vi "Close Instrument.vi"(8 "error in (no error)":errorcluster, 11 "Example Instrument in":refnum<class "LevyLab Instrument.lvclass">) -> (0 "error out":errorcluster, 3 "Example Instrument out":refnum<class "LevyLab Instrument.lvclass">)   [LabVIEW 2016, in "LevyLab Instrument.lvclass"]
uses:
  LevyLab Instrument.lvclass
  SMOs/Instrument/Instrument.lvclass
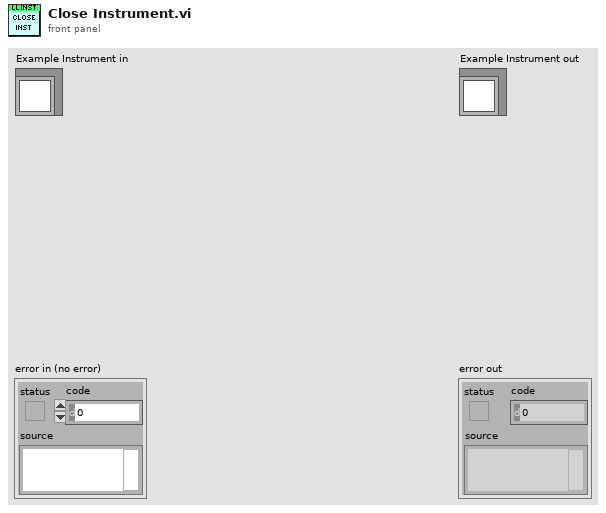
[diagram p1: front panel]
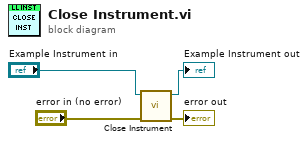
[diagram p0: block diagram]
diagram:
  n1 = call-parent "Close Instrument.vi"("error in (no error)"="error in (no error)", "Instrument in"="Example Instrument in") -> ("error out"=→"error out":errorcluster, "Instrument out"=→"Example Instrument out":refnum<class "LevyLab Instrument.lvclass">)  [unwired: 8 in]
